vi "Triggered Continuous Buffered Generation.vi"() -> ()   [LabVIEW 2009]
uses:
  <vilib>/DAQmx/write.llb/DAQmx Write (Analog Wfm 1Chan NSamp).vi
  <vilib>/DAQmx/configure/timing.llb/DAQmx Timing (Sample Clock).vi
  <vilib>/DAQmx/configure/trigger.llb/DAQmx Start Trigger (Digital Edge).vi
  <vilib>/DAQmx/create/channels.llb/DAQmx Create Channel (AO-Voltage-Basic).vi
panel:
  in  "stop":bool
  in  "physical channels":tag
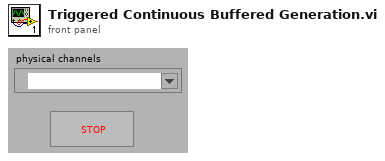
[diagram p1: front panel]
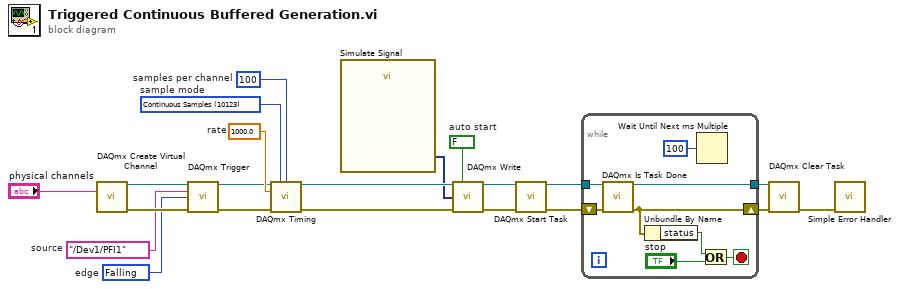
[diagram p0: block diagram]
diagram:
  w1 = 10171 items=["Rising"=10280, "Falling"=10171]  # edge
  w2 = tag "/Dev1/PFI1"  # source
  w8 = 100  # samples per channel
  w10 = 10123 items=["Finite Samples"=10178, "Continuous Samples"=10123, "Hardware Timed Single Point"=12522]  # sample mode
  w11 = FALSE  # auto start
  w21 = 1000.0  # rate
  n1 = call-poly <vilib>:"DAQmx Create Virtual Channel.vi"("physical channels"="physical channels") -> ("task out"=w4:refnum<k21>, "error out"=w6:errorcluster)  [unwired: 13 in]
  n2 = call-poly <vilib>:"DAQmx Trigger.vi"("task/channels in"=w4, "source"=w2, "edge"=w1, "error in"=w6) -> ("task out"=w3:refnum<k21>, "error out"=w5:errorcluster)  [unwired: 10 in]
  n3 = call-poly <vilib>:"DAQmx Timing.vi"("task/channels in"=w3, "sample mode"=w10, "samples per channel"=w8, "rate"=w21, "error in"=w5) -> ("task out"=w20:refnum<k21>, "error out"=w19:errorcluster)  [unwired: 9 in]
  n4 = call "Simulate Signal"() -> ("Triangle with Uniform Noise"=w7:dynamicdata)  [unwired: 14 in, 1 out]
  n5 = call-poly <vilib>:"DAQmx Write.vi"("task/channels in"=w20, "auto start"=w11, "data"=w7, "error in"=w19) -> ("task out"=w18:refnum<k21>, "error out"=w17:errorcluster)  [unwired: 9 in, 1 out]
  n6 = call <vilib>:"DAQmx Start Task.vi"("task/channels in"=w18, "error in"=w17) -> ("task out"=w16:refnum<k21>, "error out"=w15:errorcluster)  [unwired: 12 in]
  n7 = while {
    tunnel: w16 -> [w29]
    tunnel: [w27] -> w14
    shift-right: [w26] -> w13
    shift-left: w15 -> [w28]
    stop <- w23 stop-if-true
    n8 = call <vilib>:"DAQmx Is Task Done.vi"("task/channels in"=w29, "error in"=w28) -> ("task out"=w27:refnum<k21>, "error out"=w26:errorcluster)  [unwired: 11 in, 1 out]
    n9 = Unbundle By Name "Unbundle By Name"(w26) -> ("status"=w25:bool)
    n10 = Wait Until Next ms Multiple(millisecond multiple=u32 100) -> ()  [unwired: 1 out]
    n11 = Or(x=w25, y="stop") -> (x .or. y?=w23:bool)
  }
  n12 = call <vilib>:"DAQmx Clear Task.vi"("task in"=w14, "error in"=w13) -> ("error out"=w12:errorcluster)  [unwired: 13 in]
  n13 = call <vilib>:"Simple Error Handler.vi"("error in (no error)"=w12) -> ()  [unwired: 4 in, 5 out]
